vi "Trav_Axis_Correction.vi"(0 "Traverse Name":string, 1 "Axis":T1, 2 "Position input XYZ":sgl[](array[numeric])=[0.0, 0.0, 0.0] format="%.2f") -> (3 "Position":dbl[](array[numeric]), 4 "Correction":dbl[](array[numeric]), 5 "Offset Array":sgl[](array[numeric]), 6 "Error String":string)   [LabVIEW 2015]
uses:
  Route mapping/Axis.ctl
  Globals/Constants_global.vi
panel:
  out "fractional index or x":dbl
  out "In Range?":bool
  out "Data Found?":bool
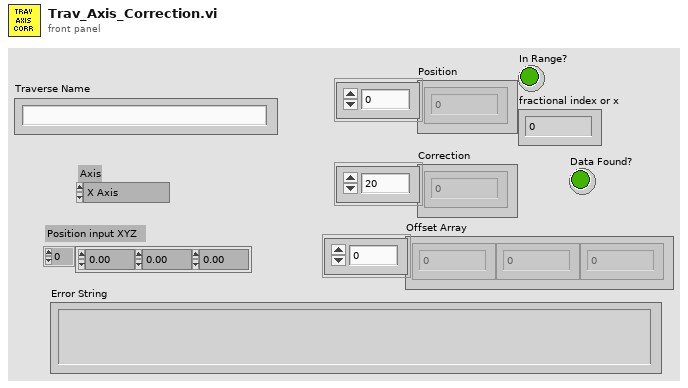
[diagram p1: front panel]
types:
  T1 = typedef "Axis.ctl" = enum16{"X Axis", "X Axis -ve", "Y Axis", "Y Axis -ve", "Z Axis", "Z Axis -ve"}
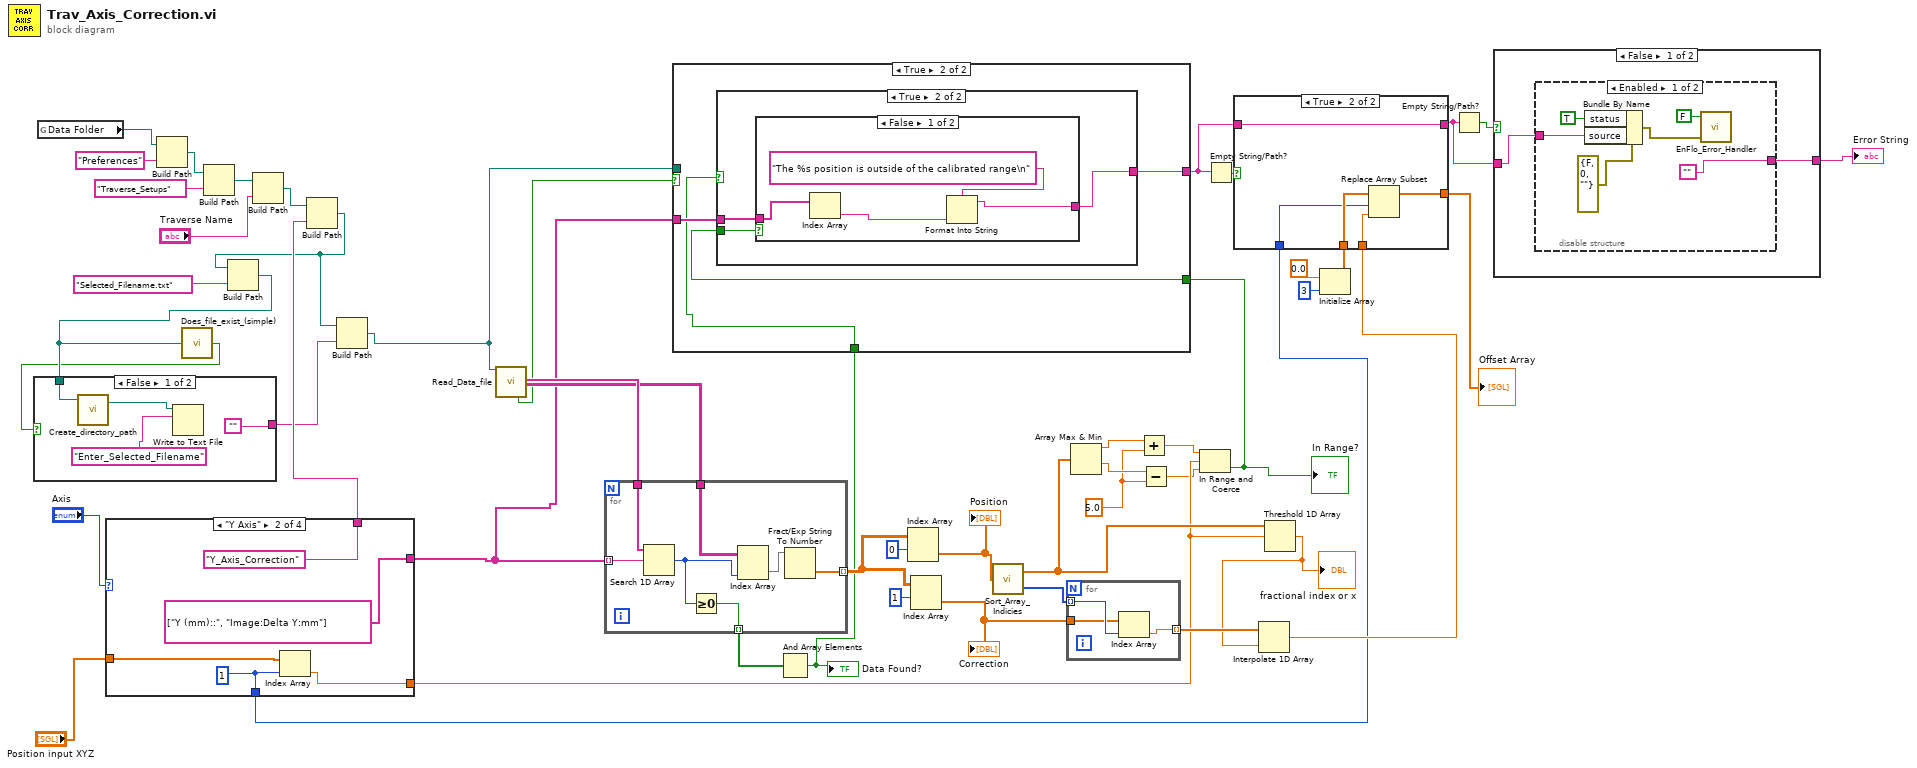
[diagram p0: block diagram]
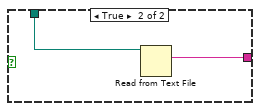
[diagram p4: hidden frame]
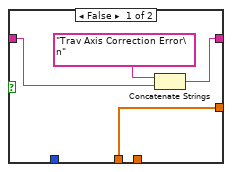
[diagram p5: hidden frame]
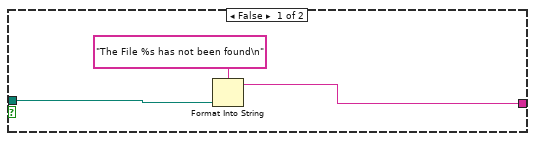
[diagram p6: hidden frame]
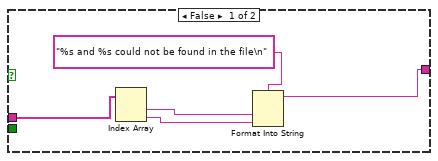
[diagram p7: hidden frame]
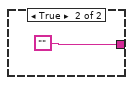
[diagram p8: hidden frame]
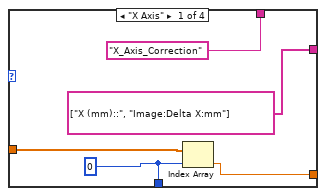
[diagram p9: hidden frame]
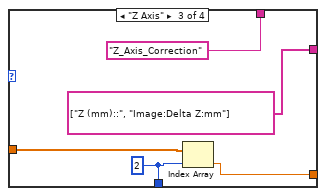
[diagram p10: hidden frame]
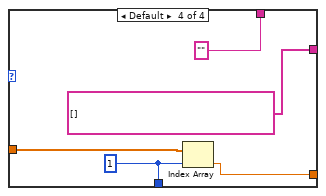
[diagram p11: hidden frame]
diagram:
  w26 = 5.0 ("y")
  n1 = global read "Constants_global.vi" "Data Folder"() -> (w48:path)
  n2 = case shown="\"Y Axis\"" "Axis" {
    tunnel: ["X_Axis_Correction" ("name or relative path") "Y_Axis_Correction" ("name or relative path") "Z_Axis_Correction" ("name or relative path") "" ("name or relative path")] -> w9
    tunnel: [string[] ["X (mm)::", "Image:Delta X:mm"] ("Ch names Out") string[] ["Y (mm)::", "Image:Delta Y:mm"] ("Ch names Out") string[] ["Z (mm)::", "Image:Delta Z:mm"] ("Ch names Out") string[] [] ("Ch names Out")] -> w20
    tunnel: "Position input XYZ" -> [w52 w57 w62 w67]
    tunnel: [w51 w56 w61 w66] -> w25
    tunnel: [w50 w55 w60 w65] -> w12
    frame "X Axis" {
      w50 = 0 ("index")
      n3 = Index Array(array=w52, index=w50) -> (element=w51:sgl)
    }
    frame "Y Axis" {
      w55 = 1 ("index")
      n4 = Index Array(array=w57, index=w55) -> (element=w56:sgl)
    }
    frame "Z Axis" {
      w60 = 2 ("index")
      n5 = Index Array(array=w62, index=w60) -> (element=w61:sgl)
    }
    frame Default {
      w65 = 1 ("index")
      n6 = Index Array(array=w67, index=w65) -> (element=w66:sgl)
    }
  }
  n7 = Build Path(base path=w48, name or relative path="Preferences") -> (appended path=w46:path)
  n8 = Build Path(base path=w46, name or relative path="Traverse_Setups") -> (appended path=w45:path)
  n9 = Build Path(base path=w45, name or relative path="Traverse Name") -> (appended path=w10:path)
  n10 = Build Path(base path=w10, name or relative path=w9) -> (appended path=w8:path)
  n11 = Build Path(base path=w8, name or relative path="Selected_Filename.txt" ("Substring")) -> (appended path=w6:path)
  n12 = call "Does_file_exist_(simple).vi"("Pathname"=w6) -> ("exists?"=w5:bool)
  n13 = case shown="False" w5 {
    tunnel: w6 -> [w72 w75]
    tunnel: ["" w74] -> w4
    frame False {
      n14 = call "Create_directory_path.vi"("Path name"=w72) -> ("Path name Out"=w71:path)  [unwired: 2 in, 1 out]
      n15 = Write to Text File(file (use dialog)=w71, text="Enter_Selected_Filename" ("Substring")) -> ()  [unwired: 2 in, 3 out]
    }
    frame True {
      n16 = Read from Text File(file (use dialog)=w75) -> (text=w74:string)  [unwired: 3 in, 3 out]
    }
  }
  n17 = Build Path(base path=w8, name or relative path=w4) -> (appended path=w7:path)
  n18 = call "Read_Data_file.vi"("Results file"=w7) -> ("EOF?"=w31:bool, "Ch names Out"=w43:string[], "Channel Values Out"=w42:string[][])  [unwired: 4 in, 12 out]
  n19 = for {
    tunnel: w43 -> [w82]
    tunnel: w20 -> [w81] mode=indexing
    tunnel: w42 -> [w80]
    tunnel: [w79] -> w39 mode=indexing
    tunnel: [w76] -> w38 mode=indexing
    n20 = Search 1D Array(1D array=w82, element=w81) -> (index of element=w77:i32)  [unwired: 1 in]
    n21 = Greater Or Equal To 0?(x=w77) -> (x >= 0?=w76:bool)
    n22 = Index Array(array=w80, index (col)=w77) -> (element=w78:string[])  [unwired: 1 in]
    n23 = Fract/Exp String To Number(string=w78) -> (number=w79:dbl[])  [unwired: 3 in, 1 out]
  }
  n24 = And Array Elements(Boolean array=w38) -> (logical AND=w21:bool)
  "Data Found?" <- w21
  n25 = Index Array(array=w39, index (row)=0) -> (element=w35:dbl[])  [unwired: 1 in]
  "Position" <- w35
  n26 = Index Array(array=w39, index (row)=1) -> (element=w33:dbl[])  [unwired: 1 in]
  "Correction" <- w33
  n27 = call "Sort_Array_Indicies.vi"("unsorted array"=w35) -> ("sorted array"=w29:dbl[], "Sort Index"=w34:i32[])
  n28 = for {
    tunnel: w34 -> [w85] mode=indexing
    tunnel: w33 -> [w84]
    tunnel: [w83] -> w32 mode=indexing
    n29 = Index Array(array=w84, index=w85) -> (element=w83:dbl)
  }
  n30 = Array Max & Min(array=w29) -> (max value=w28:dbl, min value=w27:dbl)  [unwired: 2 out]
  n31 = Add(x=w28, y=w26) -> (x+y=w24:dbl)
  n32 = Subtract(x=w27, y=w26) -> (x-y=w23:dbl)
  n33 = In Range and Coerce(upper limit=w24, x=w25, lower limit=w23) -> (In Range?=w22:bool)  [unwired: 1 out]
  "In Range?" <- w22
  n34 = case shown="True" w31 {
    tunnel: w7 -> [w88 _]
    tunnel: [w86 w91] -> w18
    tunnel: w22 -> [_ w92]
    tunnel: w20 -> [_ w90]
    tunnel: w21 -> [_ w89]
    frame False {
      n35 = Format Into String(format string="The File %s has not been found\n", w88) -> (resulting string=w86:string)  [unwired: 2 in, 1 out]
    }
    frame True {
      n36 = case shown="True" w89 {
        tunnel: w92 -> [_ w100]
        tunnel: [w93 w99] -> w91
        tunnel: w90 -> [w96 w98]
        frame False {
          n37 = Index Array(array=w96) -> (element #1=w97:string, element #2=w95:string)  [unwired: 2 in]
          n38 = Format Into String(format string="%s and %s could not be found in the file\n", w97, w95) -> (resulting string=w93:string)  [unwired: 2 in, 1 out]
        }
        frame True {
          n39 = case shown="False" w100 {
            tunnel: w98 -> [w103 _]
            tunnel: [w101 ""] -> w99
            frame False {
              n40 = Index Array(array=w103) -> (element=w102:string)  [unwired: 1 in]
              n41 = Format Into String(format string="The %s position is outside of the calibrated range\n", w102) -> (resulting string=w101:string)  [unwired: 2 in, 1 out]
            }
            frame True {
            }
          }
        }
      }
    }
  }
  n42 = Empty String/Path?(string/path=w18) -> (empty?=w19:bool)
  n43 = Threshold 1D Array(2:w25, 3:w29) -> (0:w30:dbl)  [unwired: 1 in]
  "fractional index or x" <- w30
  n44 = Interpolate 1D Array(1:w30, 2:w32) -> (0:w17:dbl)
  n45 = Initialize Array(sgl 0.0, 3 ("dimension size")) -> (w14:sgl[])
  n46 = case shown="True" w19 {
    tunnel: [w107 w114] -> w1
    tunnel: w18 -> [w109 w114]
    tunnel: w17 -> [_ w113]
    tunnel: w14 -> [w106 w112]
    tunnel: [w106 w111] -> w13
    tunnel: w12 -> [_ w110]
    frame False {
      n47 = Concatenate Strings("Trav Axis Correction Error\n" ("string"), w109) -> (w107:string)
    }
    frame True {
      n48 = Replace Array Subset(array=w112, new element=w113, index=w110) -> (w111:sgl[])
    }
  }
  "Offset Array" <- w13
  n49 = Empty String/Path?(string/path=w1) -> (empty?=w3:bool)
  n50 = case shown="False" w3 {
    tunnel: [w115 w124] -> w2
    tunnel: w1 -> [w116 w124]
    frame False {
      n51 = disable-structure shown="Enabled" {
        disable-tunnel: w116 -> [w122 w123]
        disable-tunnel: ["" w123] -> w115
        frame Enabled {
          n52 = Bundle By Name(cluster=errorcluster {"status"=FALSE, "code"=0, "source"=""} ("error in (no error)"), "status"=TRUE, "source"=w122) -> (w118:errorcluster)
          n53 = call "EnFlo_Error_Handler.vi"("error in (no error)"=w118, "Dialog Box (T)"=FALSE) -> ()  [unwired: 1 in, 3 out]
        }
        frame Disabled {
        }
      }
    }
    frame True {
    }
  }
  "Error String" <- w2
